vi "LV_AD 转换位移.vi"(5 "采样次数":i32=400, 10 "AD通道":i32) -> (2 "实际位移":dbl)   [LabVIEW 2010]
uses:
  idd.vi
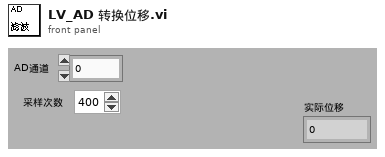
[diagram p1: front panel]
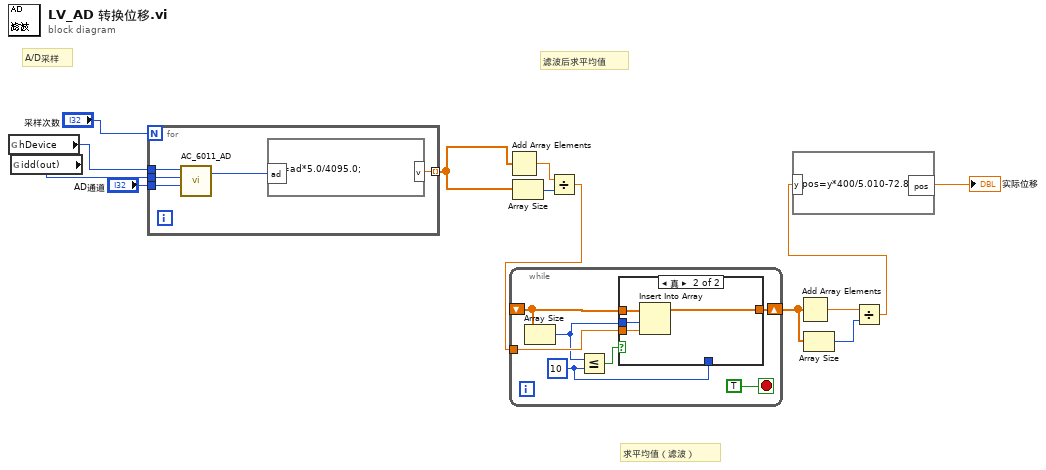
[diagram p0: block diagram]
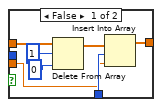
[diagram p2: hidden frame]
diagram:
  # "求平均值（滤波）"
  # "滤波后求平均值"
  # "A/D采样"
  n1 = global read "idd.vi" "hDevice"() -> (w12:u32)
  n2 = global read "idd.vi" "idd(out)"() -> (w13:u32)
  n3 = for {
    N: "采样次数" -> [_]
    tunnel: w13 -> [w18]
    tunnel: w12 -> [w17]
    tunnel: [w16] -> w7 mode=indexing
    tunnel: "AD通道" -> [w14]
    n4 = call "AC_6011_AD.vi"("ch"=w14, "idd(out)"=w18, "hDevice(in)"=w17) -> ("data"=w15:i32)  [unwired: 1 in, 1 out]
    n5 = formula code="v=ad*5.0/4095.0;"("ad"=w15) -> ("v"=w16:dbl)
  }
  n6 = Add Array Elements(numeric array=w7) -> (sum=w8:dbl)
  n7 = Array Size(array=w7) -> (size(s)=w9:i32)
  n8 = Divide(x=w8, y=w9) -> (x/y=w2:dbl)
  n9 = while {
    shift-right: [w22] -> w4
    shift-left: _ -> [w24]
    tunnel: w2 -> [w23]
    stop <- TRUE stop-if-true
    w19 = 10 ("y")
    n10 = Array Size(array=w24) -> (size(s)=w20:i32)
    n11 = Less Or Equal?(x=w20, y=w19) -> (x <= y?=w21:bool)
    n12 = case shown="真" w21 {
      tunnel: w24 -> [w32 w36]
      tunnel: w23 -> [w26 w35]
      tunnel: w20 -> [_ w34]
      tunnel: [w29 w33] -> w22
      tunnel: w19 -> [w27 _]
      frame False {
        n13 = Delete From Array(array=w32, length=1 ("长度"), index=0 ("索引")) -> (array with subset deleted=w28:dbl[])  [unwired: 1 out]
        n14 = Insert Into Array(array=w28, index=w27, new element=w26) -> (w29:dbl[])
      }
      frame True {
        n15 = Insert Into Array(array=w36, index=w34, new element=w35) -> (w33:dbl[])
      }
    }
  }
  n16 = Add Array Elements(numeric array=w4) -> (sum=w5:dbl)
  n17 = Array Size(array=w4) -> (size(s)=w3:i32)
  n18 = Divide(x=w5, y=w3) -> (x/y=w1:dbl)
  n19 = formula code="pos=y*400/5.010-72.894;"("y"=w1) -> ("pos"=→"实际位移":dbl)
